vi "Main.vi"(11 "Module Admin":refnum<class "Delacor_lib_QMH_Cloneable Module Admin.lvclass">) -> ()   [LabVIEW 2020, in "Controlador.lvlib"]
doc: "This template is based off of the Queued Message Handler design pattern and the Queued Message Handler project template that ships with LabVIEW.\n\nThe main difference is that the queue is private to this module and communication between modules is performed via Broadcast and Request events.\n\nRequest events are wrapped in public API methods and are handled in the Event Handling Loop (EHL) of this VI. Any module can register for Broadcast events sent by this module. The EHL generates messages based on user interface actions.\n\nThe Message Handling Loop (MHL) processes messages generated by the EHL, or by other messages. The messages are string values, so new messages can be added easily to the Message Cases case structure in the MHL. Each message cluster can also provide an optional value for Message Data, which is a variant that can be converted to whatever message-specific data is required.\n_____\nBased on DQMH Project Template 6.0.0.91."
uses:
  Controlador.lvlib
  <vilib>/Delacor/Delacor QMH/Libraries/Cloneable Module Admin_class/Delacor_lib_QMH_Cloneable Module Admin.lvclass
  C:/Program Files (x86)/National Instruments/LabVIEW 2020/vi.lib/Delacor/Delacor QMH/Libraries/Module Admin_class/Delacor_lib_QMH_Module Admin.lvclass
  Module Data--cluster.ctl
  Class/Osciloscope/Osciloscope.lvclass
  <vilib>/Delacor/Delacor QMH/Libraries/Message Queue_class/Delacor_lib_QMH_Message Queue.lvclass/Delacor_lib_QMH_Message Queue.ctl
  <vilib>/Delacor/Delacor QMH/Libraries/Cloneable Module Admin_class/Delacor_lib_QMH_Cloneable Module Admin.lvclass/Delacor_lib_QMH_Cloneable Module Admin.ctl
  Stop Argument--cluster.ctl
  <vilib>/Delacor/Delacor QMH/Libraries/Module Admin_class/Delacor_lib_QMH_Module Admin.lvclass/Delacor_lib_QMH_Module Admin.ctl
  Set COM Port Argument--cluster.ctl
  Initialize Osciloscope Argument--cluster.ctl
  Close Osciloscope Argument--cluster.ctl
  Autosetup Osciloscope Argument--cluster.ctl
  Configure Channel OS Argument--cluster.ctl
  Read Measurement Argument--cluster.ctl
  Read Measurement (Reply Payload)--cluster.ctl
  Read Measurement 2 Channels Argument--cluster.ctl
  Read Measurement 2 Channels (Reply Payload)--cluster.ctl
  Read Waveform Argument--cluster.ctl
  Reset Argument--cluster.ctl
  <vilib>/Utility/miscctls.llb/LVPointTypeDef.ctl
  Class/Osciloscope/Osciloscope.lvclass/Osciloscope.ctl
  <vilib>/Delacor/Delacor QMH/Libraries/Message Queue_class/Delacor_lib_QMH_Enqueue Message (Single).vi
  <vilib>/Delacor/Delacor QMH/Libraries/Cloneable Module Admin_class/Delacor_lib_QMH_Get Module ID.vi
  <vilib>/Delacor/Delacor QMH/Libraries/Module Admin_class/Delacor_lib_QMH_Get External Launch.vi
  Class/Osciloscope/Write COM.vi
  <vilib>/Utility/error.llb/Error Cluster From Error Code.vi
  <vilib>/ErrorRing/Error Ring.xnode
  <vilib>/Delacor/Delacor QMH/Libraries/Message Queue_class/Delacor_lib_QMH_Message Queue.lvclass
panel:
  out "error out":errorcluster
  out "Status":string
  in  "Simulate EHL Error":bool
  in  "Simulate MHL Error":bool
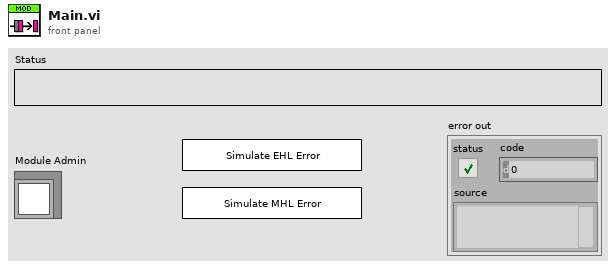
[diagram p1: front panel]
types:
  T1 = typedef "Controlador.lvlib/Request Events--cluster.ctl" = cluster{"Stop Module":refnum<user-event>, "Show Panel":refnum<user-event>, "Hide Panel":refnum<user-event>, "Show Diagram":refnum<user-event>, "Get Module Execution Status":refnum<user-event>, "Set COM Port":refnum<user-event>, "Initialize Osciloscope":refnum<user-event>, "Close Osciloscope":refnum<user-event>, "Autosetup Osciloscope":refnum<user-event>, "Configure Channel OS":refnum<user-event>, "Read Measurement":refnum<user-event>, "Read Measurement 2 Channels":refnum<user-event>, "Read Waveform":refnum<user-event>, "Reset":refnum<user-event>, "Probe":refnum<user-event>}
  T2 = typedef "Controlador.lvlib/Module Data--cluster.ctl" = cluster{"Status":string, "Osciloscope":refnum<class "Osciloscope.lvclass">}
  T3 = enum32{"invalid lock state", "Not Locked", "Locked (No Password)", "Password-protected"}
  T4 = typedef "Controlador.lvlib/Stop Argument--cluster.ctl" = cluster{"Module ID":i32, "Origin":string, "Exit via Stop Module Req?":bool, "Wait for Module to stop?":bool}
  T5 = typedef "Controlador.lvlib/Set COM Port Argument--cluster.ctl" = cluster{"Module ID":i32, "COM":refnum<visa-resource-name>}
  T6 = typedef "Controlador.lvlib/Initialize Osciloscope Argument--cluster.ctl" = cluster{"Module ID":i32, "Serial Configuration":cluster{"Baud Rate":u32, "Parity":u16, "Stop Bits":u16, "Flow Control":u16}}
  T7 = typedef "Controlador.lvlib/Close Osciloscope Argument--cluster.ctl" = cluster{"Module ID":i32, "Boolean":bool}
  T8 = typedef "Controlador.lvlib/Autosetup Osciloscope Argument--cluster.ctl" = cluster{"Module ID":i32, "Boolean":bool}
  T9 = typedef "Controlador.lvlib/Configure Channel OS Argument--cluster.ctl" = cluster{"Module ID":i32, "Config Channel":cluster{"Channel (0: Channel 1)":i32, "Vertical Coupling (1: DC)":i32, "Probe Attenuation (10: 10X)":i32, "Vertical Range (10.0 V/div)":dbl, "Vertical Offset (0.0 divs)":dbl, "Bandwidth (0: MAX Bandwidth)":i32, "Enable Channel (True)":bool}}
  T10 = typedef "Controlador.lvlib/Read Measurement Argument--cluster.ctl" = cluster{"Module ID":i32, "Wait Notifier":refnum<notifier>, "wait for reply":bool, "Measurement Type (0: Frequency)":i32, "Channel (1: Channel 1)":i32}
  T11 = typedef "Controlador.lvlib/Read Measurement 2 Channels Argument--cluster.ctl" = cluster{"Module ID":i32, "Wait Notifier":refnum<notifier>, "wait for reply":bool, "Channel 2 (2: Channel 2)":i32, "Channel 1 (1: Channel 1)":i32, "Measurement Type (0: Phase)":i32}
  T12 = typedef "Controlador.lvlib/Read Waveform Argument--cluster.ctl" = cluster{"Module ID":i32, "Boolean":bool}
  T13 = typedef "Controlador.lvlib/Reset Argument--cluster.ctl" = cluster{"Module ID":i32, "Boolean":bool}
  T14 = typedef "LVPointTypeDef.ctl" = cluster{"Horizontal":i16, "Vertical":i16}
  T15 = enum32{"Invalid", "Standard", "Closed", "Hidden", "Minimized", "Maximized"}
  T16 = typedef "Controlador.lvlib/Read Measurement (Reply Payload)--cluster.ctl" = cluster{"Read Measurement_error":errorcluster, "Units":string, "Measurement":dbl}
  T17 = typedef "Controlador.lvlib/Read Measurement 2 Channels (Reply Payload)--cluster.ctl" = cluster{"Read Measurement 2 Channels_error":errorcluster, "Units":string, "Measurement":dbl}
  T18 = cluster{"Baud Rate":u32, "Parity":u16, "Stop Bits":u16, "Flow Control":u16}
  T19 = cluster{"Channel (0: Channel 1)":i32, "Vertical Coupling (1: DC)":i32, "Probe Attenuation (10: 10X)":i32, "Vertical Range (10.0 V/div)":dbl, "Vertical Offset (0.0 divs)":dbl, "Bandwidth (0: MAX Bandwidth)":i32, "Enable Channel (True)":bool}
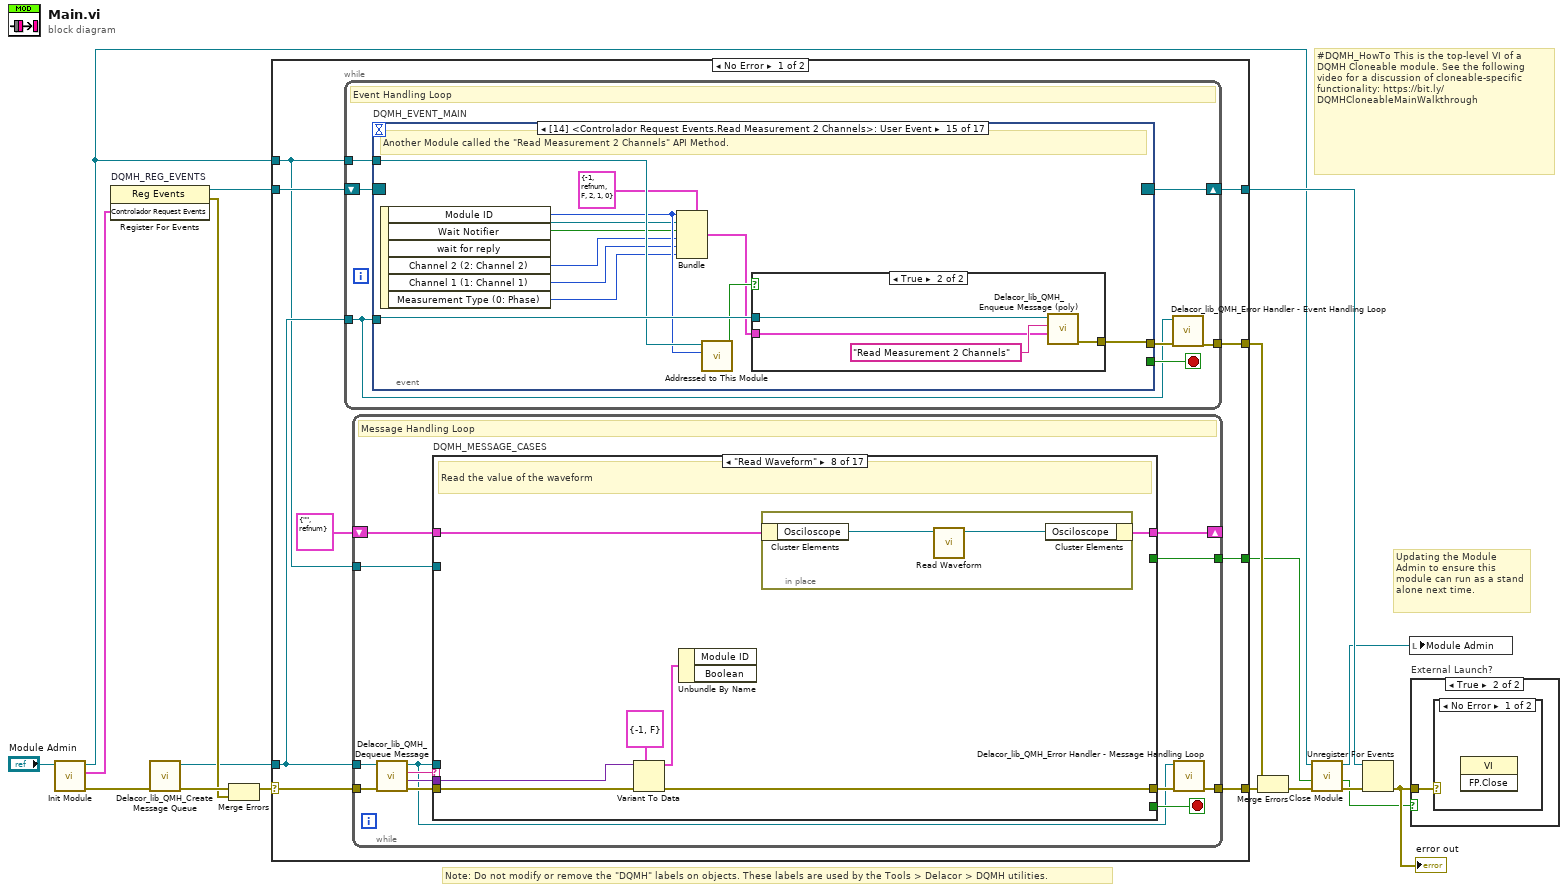
[diagram p0: block diagram]
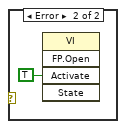
[diagram p3: hidden frame]
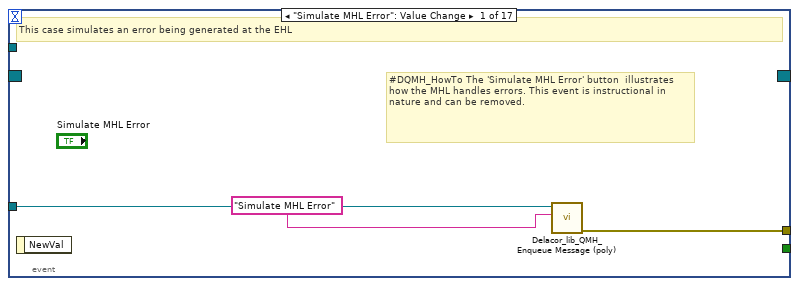
[diagram p4: hidden frame]
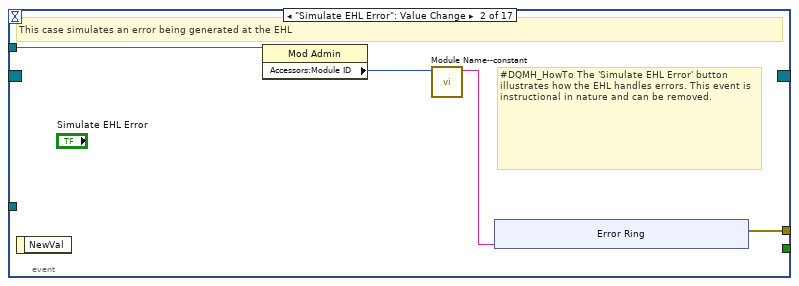
[diagram p5: hidden frame]
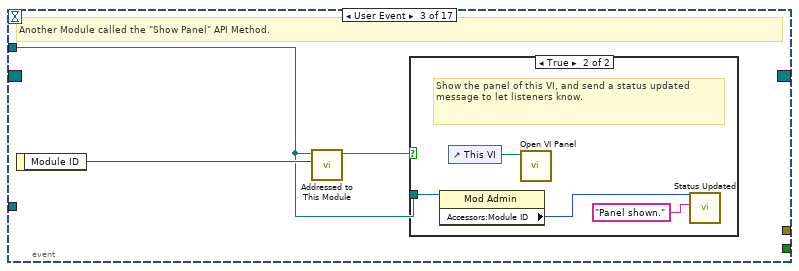
[diagram p6: hidden frame]
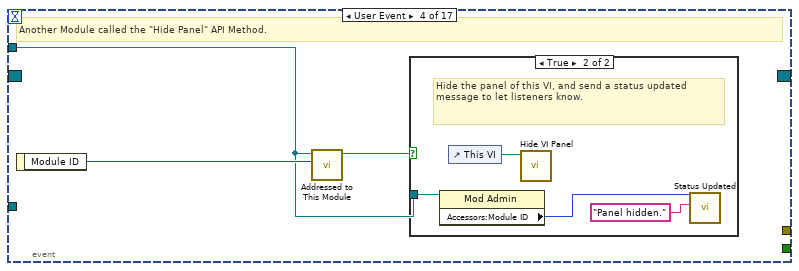
[diagram p8: hidden frame]
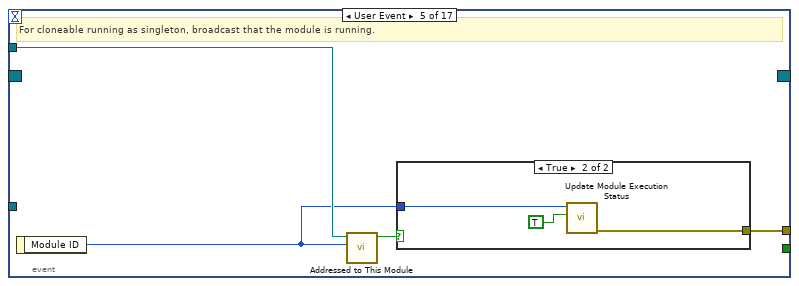
[diagram p10: hidden frame]
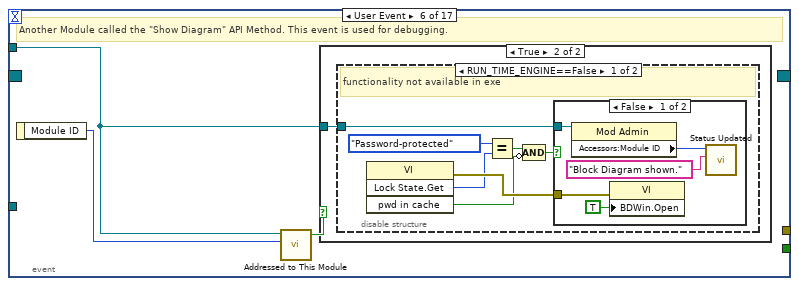
[diagram p12: hidden frame]
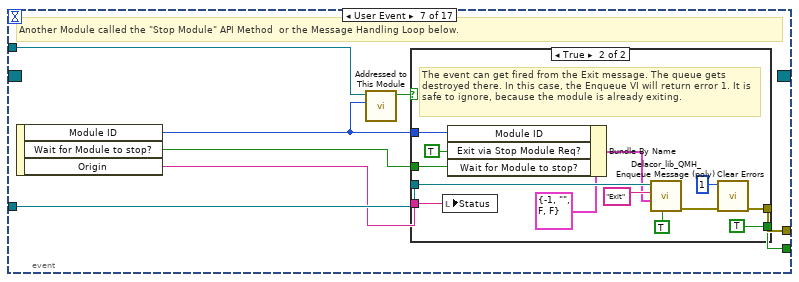
[diagram p16: hidden frame]
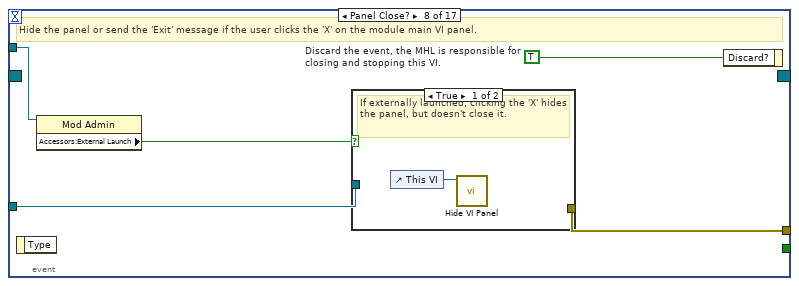
[diagram p18: hidden frame]
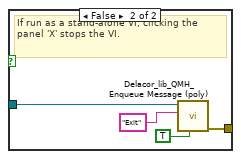
[diagram p19: hidden frame]
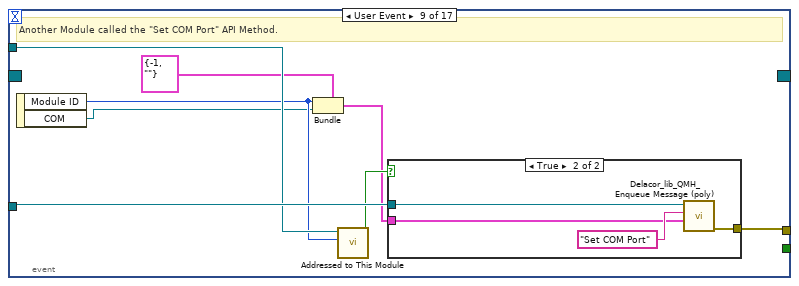
[diagram p20: hidden frame]
diagram:
  # "#DQMH_HowTo This is the top-level VI of a DQMH Cloneable module. See the following video for a discussion of cloneable-specific functionality: https://bit.ly/DQMHCloneableMainWalkthrough"
  # "Note: Do not modify or remove the \"DQMH\" labels on objects. These labels are used by the Tools > Delacor > DQMH utilities."
  # "Updating the Module Admin to ensure this module can run as a stand alone next time."
  n1 = call "Init Module.vi"("Cloneable Module Admin in"="Module Admin") -> ("error out"=w15:errorcluster, "Controlador Request Events"=w7:T1, "Cloneable Module Admin out"=w4:refnum<class "Delacor_lib_QMH_Cloneable Module Admin.lvclass">)  [unwired: 8 in]
  n2 = register-events "DQMH_REG_EVENTS"(w7) -> (reference out=w8:refnum<event-registration>, error out=w10:errorcluster)  [unwired: 2 in]
  n3 = call <vilib>:"Delacor_lib_QMH_Create Message Queue.vi"("error in"=w15) -> ("error out"=w12:errorcluster, "Message Queue"=w6:refnum<class "Delacor_lib_QMH_Message Queue.lvclass">)  [unwired: 9 in]
  n4 = Merge Errors(w12, w10) -> (w11:errorcluster)
  n5 = case shown="No Error" w11 {
    selector: w11 -> [w25 w455]
    tunnel: [w27 w454] -> w16
    tunnel: [w24 w462] -> w9
    tunnel: w8 -> [w22 w462]
    tunnel: w6 -> [w21 w453]
    tunnel: [w26 _] -> w17
    tunnel: w4 -> [w20 w458]
    tunnel: [w19 _] -> w2
    frame No Error {
      n6 = while {
        tunnel: w21 -> [w28]
        shift-right: [w31] -> w24
        shift-left: w22 -> [w32]
        tunnel: [w33] -> w26
        tunnel: w20 -> [w29]
        stop <- w30 stop-if-true
        # "Event Handling Loop"
        n7 = event "DQMH_EVENT_MAIN" shown="[14] <Controlador Request Events.Read Measurement 2 Channels>: User Event" {
          selector: w32 -> [_ _ _ _ _ _ _ _ _ _ _ _ _ _ _ _ _]
          dyn-events: [_ _ _ _ _ _ _ _ _ _ _ _ _ _ _ _ _] -> w31
          timeout: _ -> [_ _ _ _ _ _ _ _ _ _ _ _ _ _ _ _ _]
          tunnel: [_ _ _ _ _ _ w89 _ _ _ _ _ _ _ _ _ _] -> w30
          tunnel: w28 -> [w36 _ _ _ _ _ w92 w108 w124 w136 w148 w160 w172 w187 w203 w215 w227]
          tunnel: [w37 w41 _ _ w66 _ w93 w111 w117 w129 w141 w153 w165 w181 w196 w208 w220] -> w34
          tunnel: w29 -> [_ w40 w49 w56 w64 w70 w91 w109 w122 w134 w146 w158 w170 w185 w201 w213 w225]
          event "Simulate MHL Error": Value Change {
            # "#DQMH_HowTo The 'Simulate MHL Error' button  illustrates how the MHL handles errors. This event is instructional in nature and can be removed."
            # "This case simulates an error being generated at the EHL"
            n8 = event-data() -> ()  [unwired: 1 in, 1 out]
            n9 = call-poly <vilib>:"Delacor_lib_QMH_Enqueue Message (poly).vi"("Message"="Simulate MHL Error", "Message Queue in"=w36) -> ("error out"=w37:errorcluster)  [unwired: 8 in, 1 out]
          }
          event "Simulate EHL Error": Value Change {
            # "#DQMH_HowTo The 'Simulate EHL Error' button  illustrates how the EHL handles errors. This event is instructional in nature and can be removed."
            # "This case simulates an error being generated at the EHL"
            n10 = event-data() -> ()  [unwired: 1 in, 1 out]
            n11 = property class="Mod Admin"(reference=w40) -> ("Accessors:Module ID"=w39:i32)  [unwired: 1 in, 2 out]
            n12 = call "Module Name--constant.vi"("Module ID"=w39) -> ("Module Name"=w38:string)  [unwired: 10 in]
            n13 = xnode "Error Ring"("parameter 0"=w38) -> ("error out"=w41:errorcluster)
          }
          event User Event {
            # "Another Module called the \"Show Panel\" API Method."
            n14 = event-data() -> ("Module ID"=w50:i32)  [unwired: 1 in]
            n15 = call "Addressed to This Module.vi"("Module ID from Argument"=w50, "Module Admin"=w49) -> ("Addressed to this instance?"=w51:bool)  [unwired: 8 in, 1 out]
            n16 = case shown="True" w51 {
              tunnel: w49 -> [_ w53]
              frame False {
              }
              frame True {
                # "Show the panel of this VI, and send a status updated message to let listeners know."
                n17 = property class="Mod Admin"(reference=w53) -> ("Accessors:Module ID"=w52:i32)  [unwired: 1 in, 2 out]
                n18 = control-ref of="This VI"() -> (w55:refnum<vi>)
                n19 = call "Open VI Panel.vi"("VI"=w55) -> ()  [unwired: 10 in, 1 out]
                n20 = call "Status Updated.vi"("Status"="Panel shown." ("format string"), "Module ID"=w52) -> ()  [unwired: 9 in, 1 out]
              }
            }
          }
          event User Event {
            # "Another Module called the \"Hide Panel\" API Method."
            n21 = event-data() -> ("Module ID"=w57:i32)  [unwired: 1 in]
            n22 = call "Addressed to This Module.vi"("Module ID from Argument"=w57, "Module Admin"=w56) -> ("Addressed to this instance?"=w58:bool)  [unwired: 8 in, 1 out]
            n23 = case shown="True" w58 {
              tunnel: w56 -> [_ w60]
              frame False {
              }
              frame True {
                # "Hide the panel of this VI, and send a status updated message to let listeners know."
                n24 = property class="Mod Admin"(reference=w60) -> ("Accessors:Module ID"=w59:i32)  [unwired: 1 in, 2 out]
                n25 = control-ref of="This VI"() -> (w62:refnum<vi>)
                n26 = call "Hide VI Panel.vi"("VI"=w62) -> ()  [unwired: 10 in, 1 out]
                n27 = call "Status Updated.vi"("Status"="Panel hidden." ("format string"), "Module ID"=w59) -> ()  [unwired: 9 in, 1 out]
              }
            }
          }
          event User Event {
            # "For cloneable running as singleton, broadcast that the module is running."
            n28 = event-data() -> ("Module ID"=w63:i32)  [unwired: 1 in]
            n29 = call "Addressed to This Module.vi"("Module ID from Argument"=w63, "Module Admin"=w64) -> ("Addressed to this instance?"=w65:bool)  [unwired: 8 in, 1 out]
            n30 = case shown="True" w65 {
              tunnel: [_ w69] -> w66
              tunnel: w63 -> [_ w68]
              frame False {
              }
              frame True {
                n31 = call "Update Module Execution Status.vi"("Running?"=TRUE, "Module ID"=w68) -> ("error out"=w69:errorcluster)  [unwired: 9 in]
              }
            }
          }
          event User Event {
            # "Another Module called the \"Show Diagram\" API Method. This event is used for debugging."
            n32 = event-data() -> ("Module ID"=w71:i32)  [unwired: 1 in]
            n33 = call "Addressed to This Module.vi"("Module ID from Argument"=w71, "Module Admin"=w70) -> ("Addressed to this instance?"=w72:bool)  [unwired: 8 in, 1 out]
            n34 = case shown="True" w72 {
              tunnel: w70 -> [_ w73]
              frame False {
              }
              frame True {
                n35 = disable-structure shown="RUN_TIME_ENGINE==False" {
                  disable-tunnel: w73 -> [w74 _]
                  frame condition #0 (active) {
                    # "functionality not available in exe"
                    n36 = invoke class="VI" method="Lock State.Get"() -> (error out=w80:errorcluster, "Get Lock State"=w79:T3, "pwd in cache"=w76:bool)  [unwired: 4 in, 1 out]
                    n37 = Equal?(x=T3."Password-protected", y=w79) -> (x = y?=w77:bool)
                    n38 = Compound Arithmetic op=AND(w77, invert w76) -> (w75:bool)
                    n39 = case shown="False" w75 {
                      tunnel: w80 -> [w85 _]
                      tunnel: w74 -> [w82 _]
                      frame False {
                        n40 = property class="Mod Admin"(reference=w82) -> ("Accessors:Module ID"=w81:i32)  [unwired: 1 in, 2 out]
                        n41 = property class="VI"(error in=w85, "BDWin.Open"=TRUE ("Block Diagram Window:Open")) -> ()  [unwired: 1 in, 2 out]
                        n42 = call "Status Updated.vi"("Status"="Block Diagram shown." ("format string"), "Module ID"=w81) -> ()  [unwired: 9 in, 1 out]
                      }
                      frame True {
                        # "Password-protected VI, and the password is not in the cache. Do not show the diagram."
                      }
                    }
                  }
                  frame condition #1 {
                  }
                }
              }
            }
          }
          event User Event {
            # "Another Module called the \"Stop Module\" API Method  or the Message Handling Loop below."
            n43 = event-data() -> ("Module ID"=w87:i32, "Wait for Module to stop?"=w88:bool, "Origin"=w86:string)  [unwired: 1 in]
            n44 = call "Addressed to This Module.vi"("Module ID from Argument"=w87, "Module Admin"=w91) -> ("Addressed to this instance?"=w90:bool)  [unwired: 8 in, 1 out]
            n45 = case shown="True" w90 {
              tunnel: [_ w105] -> w93
              tunnel: w92 -> [_ w101]
              tunnel: [_ TRUE] -> w89
              tunnel: w88 -> [_ w96]
              tunnel: w87 -> [_ w98]
              tunnel: w86 -> [_ w94]
              frame False {
              }
              frame True {
                # "The event can get fired from the Exit message. The queue gets destroyed there. In this case, the Enqueue VI will return error 1. It is safe to ignore, because the module is already exiting."
                n46 = local write "Status"(w94) -> ()
                n47 = Bundle By Name(cluster=T4 {"Module ID"=-1, "Origin"="", "Exit via Stop Module Req?"=FALSE, "Wait for Module to stop?"=FALSE} ("Stop Argument"), "Module ID"=w98, "Exit via Stop Module Req?"=TRUE, "Wait for Module to stop?"=w96) -> (w95:T4)
                n48 = call-poly <vilib>:"Delacor_lib_QMH_Enqueue Message (poly).vi"("Priority Message? (F)"=TRUE, "Message Data"=w95, "Message"="Exit", "Message Queue in"=w101) -> ("error out"=w106:errorcluster)  [unwired: 6 in, 1 out]
                n49 = call <vilib>:"Clear Errors.vi"("error in (no error)"=w106, "specific error code to clear (0: all)"=1) -> ("error out"=w105:errorcluster)  [unwired: 4 in, 1 out]
              }
            }
          }
          event Panel Close? {
            w110 = TRUE  # Discard the event, the MHL is responsible for closing and stopping this VI.
            # "Hide the panel or send the 'Exit' message if the user clicks the 'X' on the module main VI panel."
            n50 = event-data() -> ()  [unwired: 1 in, 1 out]
            n51 = property class="Mod Admin"(reference=w109) -> ("Accessors:External Launch"=w107:bool)  [unwired: 1 in, 2 out]
            n52 = case shown="True" w107 {
              tunnel: w108 -> [_ w115]
              tunnel: [_ w116] -> w111
              frame True {
                # "If externally launched, clicking the 'X' hides the panel, but doesn't close it."
                n53 = control-ref of="This VI"() -> (w112:refnum<vi>)
                n54 = call "Hide VI Panel.vi"("VI"=w112) -> ()  [unwired: 10 in, 1 out]
              }
              frame False {
                # "If run as a stand-alone VI, clicking the panel 'X' stops the VI."
                n55 = call-poly <vilib>:"Delacor_lib_QMH_Enqueue Message (poly).vi"("Priority Message? (F)"=TRUE, "Message"="Exit", "Message Queue in"=w115) -> ("error out"=w116:errorcluster)  [unwired: 7 in, 1 out]
              }
            }
            n56 = event-data("Discard?"=w110) -> ()  [unwired: 1 in, 1 out]
          }
          event User Event {
            # "Another Module called the \"Set COM Port\" API Method."
            n57 = event-data() -> ("Module ID"=w119:i32, "COM"=w118:refnum<visa-resource-name>)  [unwired: 1 in]
            n58 = Bundle(cluster=T5 {"Module ID"=-1, "COM"=""} ("Set COM Port Argument"), "Module ID"=w119, "COM"=w118) -> (w120:T5)
            n59 = call "Addressed to This Module.vi"("Module ID from Argument"=w119, "Module Admin"=w122) -> ("Addressed to this instance?"=w123:bool)  [unwired: 8 in, 1 out]
            n60 = case shown="True" w123 {
              tunnel: w124 -> [_ w128]
              tunnel: w120 -> [_ w126]
              tunnel: [_ w125] -> w117
              frame False {
              }
              frame True {
                n61 = call-poly <vilib>:"Delacor_lib_QMH_Enqueue Message (poly).vi"("Message Data"=w126, "Message"="Set COM Port", "Message Queue in"=w128) -> ("error out"=w125:errorcluster)  [unwired: 7 in, 1 out]
              }
            }
          }
          event User Event {
            # "Another Module called the \"Initialize Osciloscope\" API Method."
            n62 = event-data() -> ("Module ID"=w131:i32, "Serial Configuration"=w130:T18)  [unwired: 1 in]
            n63 = Bundle(cluster=T6 {"Module ID"=-1, "Serial Configuration"={"Baud Rate"=9600, "Parity"=0, "Stop Bits"=10, "Flow Control"=2}} ("Initialize Osciloscope Argument"), "Module ID"=w131, "Serial Configuration"=w130) -> (w132:T6)
            n64 = call "Addressed to This Module.vi"("Module ID from Argument"=w131, "Module Admin"=w134) -> ("Addressed to this instance?"=w135:bool)  [unwired: 8 in, 1 out]
            n65 = case shown="True" w135 {
              tunnel: w136 -> [_ w140]
              tunnel: w132 -> [_ w138]
              tunnel: [_ w137] -> w129
              frame False {
              }
              frame True {
                n66 = call-poly <vilib>:"Delacor_lib_QMH_Enqueue Message (poly).vi"("Message Data"=w138, "Message"="Initialize Osciloscope", "Message Queue in"=w140) -> ("error out"=w137:errorcluster)  [unwired: 7 in, 1 out]
              }
            }
          }
          event User Event {
            # "Another Module called the \"Close Osciloscope\" API Method."
            n67 = event-data() -> ("Module ID"=w143:i32, "Boolean"=w142:bool)  [unwired: 1 in]
            n68 = Bundle(cluster=T7 {"Module ID"=-1, "Boolean"=FALSE} ("Close Osciloscope Argument"), "Module ID"=w143, "Boolean"=w142) -> (w144:T7)
            n69 = call "Addressed to This Module.vi"("Module ID from Argument"=w143, "Module Admin"=w146) -> ("Addressed to this instance?"=w147:bool)  [unwired: 8 in, 1 out]
            n70 = case shown="True" w147 {
              tunnel: w148 -> [_ w152]
              tunnel: w144 -> [_ w150]
              tunnel: [_ w149] -> w141
              frame False {
              }
              frame True {
                n71 = call-poly <vilib>:"Delacor_lib_QMH_Enqueue Message (poly).vi"("Message Data"=w150, "Message"="Close Osciloscope", "Message Queue in"=w152) -> ("error out"=w149:errorcluster)  [unwired: 7 in, 1 out]
              }
            }
          }
          event User Event {
            # "Another Module called the \"Autosetup Osciloscope\" API Method."
            n72 = event-data() -> ("Module ID"=w155:i32, "Boolean"=w154:bool)  [unwired: 1 in]
            n73 = Bundle(cluster=T8 {"Module ID"=-1, "Boolean"=FALSE} ("Autosetup Osciloscope Argument"), "Module ID"=w155, "Boolean"=w154) -> (w156:T8)
            n74 = call "Addressed to This Module.vi"("Module ID from Argument"=w155, "Module Admin"=w158) -> ("Addressed to this instance?"=w159:bool)  [unwired: 8 in, 1 out]
            n75 = case shown="True" w159 {
              tunnel: w160 -> [_ w164]
              tunnel: w156 -> [_ w162]
              tunnel: [_ w161] -> w153
              frame False {
              }
              frame True {
                n76 = call-poly <vilib>:"Delacor_lib_QMH_Enqueue Message (poly).vi"("Message Data"=w162, "Message"="Autosetup Osciloscope", "Message Queue in"=w164) -> ("error out"=w161:errorcluster)  [unwired: 7 in, 1 out]
              }
            }
          }
          event User Event {
            # "Another Module called the \"Configure Channel OS\" API Method."
            n77 = event-data() -> ("Module ID"=w167:i32, "Config Channel"=w166:T19)  [unwired: 1 in]
            n78 = Bundle(cluster=T9 {"Module ID"=-1, "Config Channel"={"Channel (0: Channel 1)"=0, "Vertical Coupling (1: DC)"=1, "Probe Attenuation (10: 10X)"=10, "Vertical Range (10.0 V/div)"=10.0, "Vertical Offset (0.0 divs)"=0.0, "Bandwidth (0: MAX Bandwidth)"=0, "Enable Channel (True)"=FALSE}} ("Configure Channel OS Argument"), "Module ID"=w167, "Config Channel"=w166) -> (w168:T9)
            n79 = call "Addressed to This Module.vi"("Module ID from Argument"=w167, "Module Admin"=w170) -> ("Addressed to this instance?"=w171:bool)  [unwired: 8 in, 1 out]
            n80 = case shown="True" w171 {
              tunnel: w172 -> [_ w176]
              tunnel: w168 -> [_ w174]
              tunnel: [_ w173] -> w165
              frame False {
              }
              frame True {
                n81 = call-poly <vilib>:"Delacor_lib_QMH_Enqueue Message (poly).vi"("Message Data"=w174, "Message"="Configure Channel OS", "Message Queue in"=w176) -> ("error out"=w173:errorcluster)  [unwired: 7 in, 1 out]
              }
            }
          }
          event User Event {
            # "Another Module called the \"Read Measurement\" API Method."
            n82 = event-data() -> ("Module ID"=w182:i32, "Wait Notifier"=w180:refnum<notifier>, "wait for reply"=w179:bool, "Measurement Type (0: Frequency)"=w178:i32, "Channel (1: Channel 1)"=w177:i32)  [unwired: 1 in]
            n83 = Bundle(cluster=T10 {"Module ID"=-1, "Wait Notifier"=refnum, "wait for reply"=FALSE, "Measurement Type (0: Frequency)"=0, "Channel (1: Channel 1)"=1} ("Read Measurement Argument"), "Module ID"=w182, "Wait Notifier"=w180, "wait for reply"=w179, "Measurement Type (0: Frequency)"=w178, "Channel (1: Channel 1)"=w177) -> (w183:T10)
            n84 = call "Addressed to This Module.vi"("Module ID from Argument"=w182, "Module Admin"=w185) -> ("Addressed to this instance?"=w186:bool)  [unwired: 8 in, 1 out]
            n85 = case shown="True" w186 {
              tunnel: w187 -> [_ w191]
              tunnel: w183 -> [_ w189]
              tunnel: [_ w188] -> w181
              frame False {
              }
              frame True {
                n86 = call-poly <vilib>:"Delacor_lib_QMH_Enqueue Message (poly).vi"("Message Data"=w189, "Message"="Read Measurement", "Message Queue in"=w191) -> ("error out"=w188:errorcluster)  [unwired: 7 in, 1 out]
              }
            }
          }
          event User Event {
            # "Another Module called the \"Read Measurement 2 Channels\" API Method."
            n87 = event-data() -> ("Module ID"=w198:i32, "Wait Notifier"=w197:refnum<notifier>, "wait for reply"=w195:bool, "Channel 2 (2: Channel 2)"=w194:i32, "Channel 1 (1: Channel 1)"=w193:i32, "Measurement Type (0: Phase)"=w192:i32)  [unwired: 1 in]
            n88 = Bundle(cluster=T11 {"Module ID"=-1, "Wait Notifier"=refnum, "wait for reply"=FALSE, "Channel 2 (2: Channel 2)"=2, "Channel 1 (1: Channel 1)"=1, "Measurement Type (0: Phase)"=0} ("Read Measurement 2 Channels Argument"), "Module ID"=w198, "Wait Notifier"=w197, "wait for reply"=w195, "Channel 2 (2: Channel 2)"=w194, "Channel 1 (1: Channel 1)"=w193, "Measurement Type (0: Phase)"=w192) -> (w199:T11)
            n89 = call "Addressed to This Module.vi"("Module ID from Argument"=w198, "Module Admin"=w201) -> ("Addressed to this instance?"=w202:bool)  [unwired: 8 in, 1 out]
            n90 = case shown="True" w202 {
              tunnel: w203 -> [_ w207]
              tunnel: w199 -> [_ w205]
              tunnel: [_ w204] -> w196
              frame False {
              }
              frame True {
                n91 = call-poly <vilib>:"Delacor_lib_QMH_Enqueue Message (poly).vi"("Message Data"=w205, "Message"="Read Measurement 2 Channels", "Message Queue in"=w207) -> ("error out"=w204:errorcluster)  [unwired: 7 in, 1 out]
              }
            }
          }
          event User Event {
            # "Another Module called the \"Read Waveform\" API Method."
            n92 = event-data() -> ("Module ID"=w210:i32, "Boolean"=w209:bool)  [unwired: 1 in]
            n93 = Bundle(cluster=T12 {"Module ID"=-1, "Boolean"=FALSE} ("Read Waveform Argument"), "Module ID"=w210, "Boolean"=w209) -> (w211:T12)
            n94 = call "Addressed to This Module.vi"("Module ID from Argument"=w210, "Module Admin"=w213) -> ("Addressed to this instance?"=w214:bool)  [unwired: 8 in, 1 out]
            n95 = case shown="True" w214 {
              tunnel: w215 -> [_ w219]
              tunnel: w211 -> [_ w217]
              tunnel: [_ w216] -> w208
              frame False {
              }
              frame True {
                n96 = call-poly <vilib>:"Delacor_lib_QMH_Enqueue Message (poly).vi"("Message Data"=w217, "Message"="Read Waveform", "Message Queue in"=w219) -> ("error out"=w216:errorcluster)  [unwired: 7 in, 1 out]
              }
            }
          }
          event User Event {
            # "Another Module called the \"Reset\" API Method."
            n97 = event-data() -> ("Module ID"=w222:i32, "Boolean"=w221:bool)  [unwired: 1 in]
            n98 = Bundle(cluster=T13 {"Module ID"=-1, "Boolean"=FALSE} ("Reset Argument"), "Module ID"=w222, "Boolean"=w221) -> (w223:T13)
            n99 = call "Addressed to This Module.vi"("Module ID from Argument"=w222, "Module Admin"=w225) -> ("Addressed to this instance?"=w226:bool)  [unwired: 8 in, 1 out]
            n100 = case shown="True" w226 {
              tunnel: w227 -> [_ w231]
              tunnel: w223 -> [_ w229]
              tunnel: [_ w228] -> w220
              frame False {
              }
              frame True {
                n101 = call-poly <vilib>:"Delacor_lib_QMH_Enqueue Message (poly).vi"("Message Data"=w229, "Message"="Reset", "Message Queue in"=w231) -> ("error out"=w228:errorcluster)  [unwired: 7 in, 1 out]
              }
            }
          }
        }
        n102 = call-dynamic "Delacor_lib_QMH_Error Handler - Event Handling Loop.vi"("error in"=w34, "Message Queue in"=w28) -> ("dup error in"=w33:errorcluster)  [unwired: 8 in, 1 out]
      }
      n103 = while {
        tunnel: w21 -> [w235]
        shift-right: [w239] -> _
        shift-left: T2 {"Status"="", "Osciloscope"=refnum} ("Data Cluster") -> [w240]
        tunnel: w25 -> [w243]
        tunnel: [w241] -> w27
        tunnel: w20 -> [w233]
        tunnel: [w232] -> w19
        stop <- w238 stop-if-true
        # "Message Handling Loop"
        n104 = call-dynamic "Delacor_lib_QMH_Dequeue Message.vi"("error in"=w243, "Message Queue in"=w235) -> ("error out"=w242:errorcluster, "Message Data"=w236:variant, "Message"=w237:string, "Message Queue out"=w234:refnum<class "Delacor_lib_QMH_Message Queue.lvclass">)  [unwired: 6 in]
        n105 = case "DQMH_MESSAGE_CASES" shown="\"Read Waveform\"" w237 {
          selector: w237 -> [_ _ _ _ _ _ _ _ _ _ _ _ _ _ _ _ w440]
          tunnel: w234 -> [_ _ _ _ _ _ _ _ _ _ _ _ _ w391 _ w430 _]
          tunnel: w242 -> [w263 w267 w275 w286 w296 w305 w315 w325 w334 w351 w375 w387 w389 w400 w413 w436 w442]
          tunnel: [w261 w267 w274 w285 w295 w304 w314 w324 w333 w350 w374 w386 w389 w396 w412 w433 w443] -> w244
          tunnel: w240 -> [w254 w266 w270 w281 w291 w300 w310 w319 w328 w342 w365 w385 w388 w395 w410 w429 w441]
          tunnel: [w253 w266 w269 w280 w290 w299 w309 w320 w329 w341 w366 w385 w388 w395 w410 w429 w441] -> w239
          tunnel: [_ _ _ _ _ _ _ _ _ _ _ _ _ _ _ w428 _] -> w238
          tunnel: w236 -> [_ _ w273 w284 w294 w303 w313 w323 w332 w349 w373 _ _ w394 _ w426 _]
          tunnel: w233 -> [w248 _ _ _ _ _ _ _ _ _ _ _ _ w393 w408 w422 w438]
          tunnel: [_ _ _ _ _ _ _ _ _ _ _ _ _ _ _ w424 _] -> w232
          frame "Initialize" {
            w245 = "Initial Message" ("Initial Message")
            # "#CodeNeeded - Initialize the appearance of the front panel."
            # "#CodeNeeded - Initialize your state data here."
            # "Initialize - Any operation that needs to be done before the module can receive messages. Synchronize Caller Events.vi will inform Start Module.vi that the module has launched and is ready to receive messages. Module Did Init.vi will broadcast that the module initialized."
            n106 = call "Synchronize Caller Events.vi"("error in (no error)"=w263, "Module Admin"=w248) -> ("error out"=w262:errorcluster, "Module Admin out"=w247:refnum<class "Delacor_lib_QMH_Cloneable Module Admin.lvclass">)  [unwired: 8 in]
            n107 = property class="Mod Admin"(reference=w247) -> ("Accessors:Module ID"=w250:i32, "Accessors:External Launch"=w249:bool)  [unwired: 1 in, 2 out]
            n108 = call "Module Name--constant.vi"("Module ID"=w250) -> ("Module Name"=w258:string)  [unwired: 10 in]
            n109 = property class="VI"("Front Panel.Title"=w258) -> (reference out=w260:refnum<vi>, error out=w265:errorcluster)  [unwired: 2 in]
            n110 = Select(t=T15."Hidden" ("State"), s=w249, f=T15."Standard" ("State")) -> (s? t:f=w255:T15)
            n111 = invoke class="VI" method="FP.Open"(reference=w260, error in=w265, "State"=w255) -> (reference out=w259:refnum<vi>, error out=w264:errorcluster)  [unwired: 2 in, 3 out]
            n112 = call "Module Name--constant.vi"("Module ID"=w250) -> ("Module Name"=w251:string)  [unwired: 10 in]
            n113 = Bundle By Name(cluster=w254, "Status"=w245) -> (w253:T2)
            n114 = invoke class="VI" method="FP.Center"(reference=w259, error in=w264) -> ()  [unwired: 1 in, 3 out]
            n115 = property on="Pane" class="Pane"("Origin"=T14 {"Horizontal"=0, "Vertical"=0}) -> ()  [unwired: 2 in, 2 out]
            n116 = call "Module Did Init.vi"("error in (no error)"=w262, "Initialized?"=TRUE, "Origin"=w251, "Module ID"=w250) -> ("error out"=w261:errorcluster)  [unwired: 7 in]
            "Status" <- w245
          }
          frame "---Module Specific---" {
            # "Separator -- The following cases handle messages specific to this Module."
          }
          frame "Set COM Port" {
            # "Set The Visa COM Port"
            n117 = Variant To Data(error in=w275, type=T5 {"Module ID"=-1, "COM"=""} ("Set COM Port Argument"), Variant=w273) -> (data=w271:T5, error out=w274:errorcluster)
            n118 = Unbundle By Name(w271) -> ("COM"=w268:refnum<visa-resource-name>)  [unwired: 1 out]
            n119 = in-place {
              in-place-border: w268 -> [w276]
              n120 = in-place-cluster #1(w270) -> ("Osciloscope"=w278:refnum<class "Osciloscope.lvclass">)
              n121 = property class="Osciloscope.lvclass"(reference=w278, "Accessors:COM"=w276) -> (reference out=w277:refnum<class "Osciloscope.lvclass">)  [unwired: 1 in, 1 out]
              n122 = in-place-cluster #1("Osciloscope"=w277) -> (w269:T2)
            }
          }
          frame "Initialize Osciloscope" {
            # "Initialize the Osciloscope instance"
            n123 = Variant To Data(error in=w286, type=T6 {"Module ID"=-1, "Serial Configuration"={"Baud Rate"=9600, "Parity"=0, "Stop Bits"=10, "Flow Control"=2}} ("Initialize Osciloscope Argument"), Variant=w284) -> (data=w282:T6, error out=w285:errorcluster)
            n124 = Unbundle By Name(w282) -> ("Serial Configuration"=w279:T18)  [unwired: 1 out]
            n125 = in-place {
              in-place-border: w279 -> [w287]
              n126 = in-place-cluster #2(w281) -> ("Osciloscope"=w289:refnum<class "Osciloscope.lvclass">)
              n127 = call-dynamic "Initialize.vi"("Serial Configuration"=w287, "Osciloscope in"=w289) -> ("Osciloscope out"=w288:refnum<class "Osciloscope.lvclass">)  [unwired: 8 in, 1 out]
              n128 = in-place-cluster #2("Osciloscope"=w288) -> (w280:T2)
            }
          }
          frame "Close Osciloscope" {
            # "Close all the activity with the osciloscope"
            n129 = Variant To Data(error in=w296, type=T7 {"Module ID"=-1, "Boolean"=FALSE} ("Close Osciloscope Argument"), Variant=w294) -> (data=w292:T7, error out=w295:errorcluster)
            n130 = Unbundle By Name(w292) -> ()  [unwired: 2 out]
            n131 = in-place {
              n132 = in-place-cluster #3(w291) -> ("Osciloscope"=w298:refnum<class "Osciloscope.lvclass">)
              n133 = call-dynamic "Close.vi"("Osciloscope in"=w298) -> ("Osciloscope out"=w297:refnum<class "Osciloscope.lvclass">)  [unwired: 9 in, 1 out]
              n134 = in-place-cluster #3("Osciloscope"=w297) -> (w290:T2)
            }
          }
          frame "Autosetup Osciloscope" {
            # "Autosetup"
            n135 = Variant To Data(error in=w305, type=T8 {"Module ID"=-1, "Boolean"=FALSE} ("Autosetup Osciloscope Argument"), Variant=w303) -> (data=w301:T8, error out=w304:errorcluster)
            n136 = Unbundle By Name(w301) -> ()  [unwired: 2 out]
            n137 = in-place {
              n138 = in-place-cluster #4(w300) -> ("Osciloscope"=w307:refnum<class "Osciloscope.lvclass">)
              n139 = call-dynamic "Autosetup.vi"("Osciloscope in"=w307) -> ("Osciloscope out"=w306:refnum<class "Osciloscope.lvclass">)  [unwired: 9 in, 1 out]
              n140 = in-place-cluster #4("Osciloscope"=w306) -> (w299:T2)
            }
          }
          frame "Configure Channel OS" {
            # "Configure the channel in the osciloscope"
            n141 = Variant To Data(error in=w315, type=T9 {"Module ID"=-1, "Config Channel"={"Channel (0: Channel 1)"=0, "Vertical Coupling (1: DC)"=1, "Probe Attenuation (10: 10X)"=10, "Vertical Range (10.0 V/div)"=10.0, "Vertical Offset (0.0 divs)"=0.0, "Bandwidth (0: MAX Bandwidth)"=0, "Enable Channel (True)"=FALSE}} ("Configure Channel OS Argument"), Variant=w313) -> (data=w311:T9, error out=w314:errorcluster)
            n142 = Unbundle By Name(w311) -> ("Config Channel"=w308:T19)  [unwired: 1 out]
            n143 = in-place {
              in-place-border: w308 -> [w316]
              n144 = in-place-cluster #5(w310) -> ("Osciloscope"=w318:refnum<class "Osciloscope.lvclass">)
              n145 = call-dynamic "Configure Channel.vi"("Config Channel"=w316, "Osciloscope in"=w318) -> ("Osciloscope out"=w317:refnum<class "Osciloscope.lvclass">)  [unwired: 8 in, 1 out]
              n146 = in-place-cluster #5("Osciloscope"=w317) -> (w309:T2)
            }
          }
          frame "Read Waveform" {
            # "Read the value of the waveform"
            n147 = Variant To Data(error in=w325, type=T12 {"Module ID"=-1, "Boolean"=FALSE} ("Read Waveform Argument"), Variant=w323) -> (data=w321:T12, error out=w324:errorcluster)
            n148 = Unbundle By Name(w321) -> ()  [unwired: 2 out]
            n149 = in-place {
              n150 = in-place-cluster #6(w319) -> ("Osciloscope"=w327:refnum<class "Osciloscope.lvclass">)
              n151 = call-dynamic "Read Waveform.vi"("Osciloscope in"=w327) -> ("Osciloscope out"=w326:refnum<class "Osciloscope.lvclass">)  [unwired: 8 in, 2 out]
              n152 = in-place-cluster #6("Osciloscope"=w326) -> (w320:T2)
            }
          }
          frame "Reset" {
            # "Reset methode"
            n153 = Variant To Data(error in=w334, type=T13 {"Module ID"=-1, "Boolean"=FALSE} ("Reset Argument"), Variant=w332) -> (data=w330:T13, error out=w333:errorcluster)
            n154 = Unbundle By Name(w330) -> ()  [unwired: 2 out]
            n155 = in-place {
              n156 = in-place-cluster #7(w328) -> ("Osciloscope"=w336:refnum<class "Osciloscope.lvclass">)
              n157 = call-dynamic "Reset.vi"("Osciloscope in"=w336) -> ("Osciloscope out"=w335:refnum<class "Osciloscope.lvclass">)  [unwired: 9 in, 1 out]
              n158 = in-place-cluster #7("Osciloscope"=w335) -> (w329:T2)
            }
          }
          frame "Read Measurement" {
            # "Read measurement 1 channel"
            n159 = Variant To Data(error in=w351, type=T10 {"Module ID"=-1, "Wait Notifier"=refnum, "wait for reply"=FALSE, "Measurement Type (0: Frequency)"=0, "Channel (1: Channel 1)"=1} ("Read Measurement Argument"), Variant=w349) -> (data=w347:T10, error out=w350:errorcluster)
            n160 = Unbundle By Name(w347) -> ("Measurement Type (0: Frequency)"=w340:i32, "Channel (1: Channel 1)"=w339:i32, "Wait Notifier"=w346:refnum<notifier>, "wait for reply"=w345:bool)
            n161 = in-place {
              in-place-border: w340 -> [w355]
              in-place-border: w339 -> [w354]
              in-place-border: [w353] -> w338
              in-place-border: [w352] -> w337
              n162 = in-place-cluster #8(w342) -> ("Osciloscope"=w357:refnum<class "Osciloscope.lvclass">)
              n163 = call-dynamic "Read Measurement.vi"("Channel (1: Channel 1)"=w354, "Measurement Type (0: Frequency)"=w355, "Osciloscope in"=w357) -> ("Measurement"=w353:dbl, "Units"=w352:string, "Osciloscope out"=w356:refnum<class "Osciloscope.lvclass">)  [unwired: 5 in, 1 out]
              n164 = in-place-cluster #8("Osciloscope"=w356) -> (w341:T2)
            }
            n165 = Bundle By Name(cluster=T16 {"Read Measurement_error"={"status"=FALSE, "code"=0, "source"=""}, "Units"="", "Measurement"=0.0} ("Read Measurement (Reply Payload)"), "Units"=w337, "Measurement"=w338) -> (w344:T16)
            n166 = case shown="True" w345 {
              tunnel: w346 -> [_ w359]
              tunnel: w344 -> [_ w358]
              frame False {
              }
              frame True {
                n167 = Send Notification(notification=w358, notifier=w359) -> ()  [unwired: 1 in, 2 out]
              }
            }
          }
          frame "Read Measurement 2 Channels" {
            n168 = Variant To Data(error in=w375, type=T11 {"Module ID"=-1, "Wait Notifier"=refnum, "wait for reply"=FALSE, "Channel 2 (2: Channel 2)"=2, "Channel 1 (1: Channel 1)"=1, "Measurement Type (0: Phase)"=0} ("Read Measurement 2 Channels Argument"), Variant=w373) -> (data=w371:T11, error out=w374:errorcluster)
            n169 = Unbundle By Name(w371) -> ("Channel 1 (1: Channel 1)"=w364:i32, "Channel 2 (2: Channel 2)"=w363:i32, "Measurement Type (0: Phase)"=w362:i32, "Wait Notifier"=w370:refnum<notifier>, "wait for reply"=w369:bool)
            n170 = in-place {
              in-place-border: w364 -> [w380]
              in-place-border: w363 -> [w379]
              in-place-border: w362 -> [w378]
              in-place-border: [w377] -> w361
              in-place-border: [w376] -> w360
              n171 = in-place-cluster #9(w365) -> ("Osciloscope"=w382:refnum<class "Osciloscope.lvclass">)
              n172 = call-dynamic "Read Measurement 2 Channels.vi"("Measurement Type (0: Phase)"=w378, "Channel 2 (2: Channel 2)"=w379, "Channel 1 (1: Channel 1)"=w380, "Osciloscope in"=w382) -> ("Measurement"=w376:dbl, "Units"=w377:string, "Osciloscope out"=w381:refnum<class "Osciloscope.lvclass">)  [unwired: 4 in, 1 out]
              n173 = in-place-cluster #9("Osciloscope"=w381) -> (w366:T2)
            }
            n174 = Bundle By Name(cluster=T17 {"Read Measurement 2 Channels_error"={"status"=FALSE, "code"=0, "source"=""}, "Units"="", "Measurement"=0.0} ("Read Measurement 2 Channels (Reply Payload)"), "Units"=w361, "Measurement"=w360) -> (w368:T17)
            n175 = case shown="True" w369 {
              tunnel: w370 -> [_ w384]
              tunnel: w368 -> [_ w383]
              frame False {
              }
              frame True {
                n176 = Send Notification(notification=w383, notifier=w384) -> ()  [unwired: 1 in, 2 out]
              }
            }
          }
          frame "---Copy This Frame---" {
            # "Duplicate this frame when creating new messages.  Change this comment in the duplicated frame to describe this message."
            n177 = Merge Errors(w387) -> (w386:errorcluster)
          }
          frame "---Exit and Error Handling---" {
            # "Separator - the following cases handle errors and exit messages."
          }
          frame "Error" {
            # "#CodeRecommended - If you ever change the name of this \"Error\" message, you'll need to update the name in the Check Loop Error.vi as well."
            # "#CodeRecommended - If the module is running in standalone mode (External Launch = FALSE), this code will pop up an error dialog and call the 'Exit' message if an error occurs. Add more fine-grained error handling here."
            # "Error - Check the error message data and respond accordingly. This message is sent by the \"Error Handler\" VIs at the end of each loop in this application."
            n178 = property class="Mod Admin"(reference=w393) -> ("Accessors:External Launch"=w392:bool, "Accessors:Module ID"=w390:i32)  [unwired: 1 in, 2 out]
            n179 = Variant To Data(error in=w400, type=errorcluster {"status"=FALSE, "code"=0, "source"=""} ("error constant"), Variant=w394) -> (data=w401:errorcluster, error out=w398:errorcluster)
            n180 = call "Error Reported.vi"("Error"=w401, "Module ID"=w390) -> ()  [unwired: 9 in, 1 out]
            n181 = case shown="False" w392 {
              tunnel: [w406 _] -> w397
              tunnel: w391 -> [w404 _]
              tunnel: w401 -> [w405 _]
              frame False {
                # "If the module is running standalone, then pop up an error dialog and call the \"Exit\" message."
                n182 = call <vilib>:"Simple Error Handler.vi"("error in (no error)"=w405) -> ()  [unwired: 4 in, 5 out]
                n183 = call-poly <vilib>:"Delacor_lib_QMH_Enqueue Message (poly).vi"("Priority Message? (F)"=TRUE, "Message"="Exit", "Message Queue in"=w404) -> ("error out"=w406:errorcluster)  [unwired: 7 in, 1 out]
              }
              frame True {
                # "If the module was launched externally, calling the Error Reported broadcast VI is the only action performed by the \"Error\" message. The module's caller can then process the error appropriately."
              }
            }
            n184 = Merge Errors(w398, w397) -> (w396:errorcluster)
            n185 = local write "error out"(w396) -> ()
          }
          frame "Simulate MHL Error" {
            # "#DQMH_HowTo The 'Simulate MHL Error' button  illustrates how the MHL handles errors. This event is instructional in nature and can be removed."
            # "Simulate an error occurring at the MHL"
            n186 = property class="Mod Admin"(reference=w408) -> ("Accessors:Module ID"=w409:i32)  [unwired: 1 in, 2 out]
            n187 = call "Module Name--constant.vi"("Module ID"=w409) -> ("Module Name"=w407:string)  [unwired: 10 in]
            n188 = xnode "Error Ring"("parameter 0"=w407) -> ("error out"=w411:errorcluster)
            n189 = Merge Errors(w413, w411) -> (w412:errorcluster)
          }
          frame "Exit" {
            w427 = 91  # 91: not all Exit messages will have an argument
            w428 = TRUE  # Stop the VI
            # "Release the message queue reference"
            # "#CodeNeeded - Add any required cleanup code here."
            # "Exit - Exit the application."
            n190 = Variant To Data(error in=w436, type=T4 {"Module ID"=-1, "Origin"="", "Exit via Stop Module Req?"=FALSE, "Wait for Module to stop?"=FALSE} ("Stop Argument"), Variant=w426) -> (data=w423:T4, error out=w431:errorcluster)
            n191 = call <vilib>:"Clear Errors.vi"("error in (no error)"=w431, "specific error code to clear (0: all)"=w427) -> ("error out"=w435:errorcluster)  [unwired: 4 in, 1 out]
            n192 = control-ref of="This VI"() -> (w421:refnum<vi>)
            n193 = call-dynamic "Delacor_lib_QMH_Release Message Queue.vi"("error in"=w435, "Message Queue"=w430) -> ("error out"=w434:errorcluster)  [unwired: 9 in]
            n194 = call "Handle Exit.vi"("Stop Argument"=w423, "Module Admin in"=w422, "VI reference"=w421) -> ("error out"=w432:errorcluster, "Wait for Stop?"=w424:bool)  [unwired: 7 in]
            n195 = Merge Errors(w434, w432) -> (w433:errorcluster)
          }
          frame Default {
            # "'Default' case only runs if there is a message that isn't defined in any of the other cases.  Output a programming error."
            n196 = property class="Mod Admin"(reference=w438) -> ("Accessors:Module ID"=w437:i32)  [unwired: 1 in, 2 out]
            n197 = call "Module Name--constant.vi"("Module ID"=w437) -> ("Module Name"=w439:string)  [unwired: 10 in]
            n198 = xnode "Error Ring"("parameter 0"=w440, "parameter 1"=w439) -> ("error out"=w444:errorcluster)
            n199 = Merge Errors(w442, w444) -> (w443:errorcluster)
          }
        }
        n200 = call-dynamic "Delacor_lib_QMH_Error Handler - Message Handling Loop.vi"("error in"=w244, "Message Queue in"=w234) -> ("dup error in"=w241:errorcluster)  [unwired: 8 in, 1 out]
      }
    }
    frame Error {
      n201 = call "Synchronize Caller Events.vi"("Module Admin"=w458) -> ("Module Admin out"=w457:refnum<class "Delacor_lib_QMH_Cloneable Module Admin.lvclass">)  [unwired: 9 in, 1 out]
      n202 = property class="Mod Admin"(reference=w457) -> ("Accessors:Module ID"=w456:i32)  [unwired: 1 in, 2 out]
      n203 = call-dynamic "Delacor_lib_QMH_Release Message Queue.vi"("error in"=w455, "Message Queue"=w453) -> ("error out"=w454:errorcluster)  [unwired: 9 in]
      n204 = call "Module Name--constant.vi"("Module ID"=w456) -> ("Module Name"=w461:string)  [unwired: 10 in]
      n205 = Format Into String(format string="An error occurred during initialization. %s is no longer running.", w461) -> (resulting string=w459:string)  [unwired: 2 in, 1 out]
      n206 = call "Error Reported.vi"("Additional Information"=w459, "Error"=w454, "Module ID"=w456) -> ()  [unwired: 8 in, 1 out]
    }
  }
  n207 = Merge Errors(w17, w16) -> (w18:errorcluster)
  n208 = call "Close Module.vi"("error in"=w18, "Wait for stop?"=w2, "Module Admin in"=w4) -> ("error out"=w14:errorcluster, "External Launch"=w1:bool, "Module Admin out"=w3:refnum<class "Delacor_lib_QMH_Cloneable Module Admin.lvclass">)  [unwired: 6 in]
  n209 = Unregister For Events(event registration refnum=w9, error in=w14) -> (error out=w13:errorcluster)
  "error out" <- w13
  n210 = local write "Module Admin"(w3) -> ()
  n211 = case "External Launch?" shown="True" w1 {
    tunnel: w13 -> [_ w463]
    frame False {
    }
    frame True {
      n212 = case shown="No Error" w463 {
        frame No Error {
          n213 = invoke class="VI" method="FP.Close"() -> ()  [unwired: 3 in, 3 out]
        }
        frame Error {
          n214 = invoke class="VI" method="FP.Open"("Activate"=TRUE ("Activate?")) -> ()  [unwired: 4 in, 5 out]
        }
      }
    }
  }
